vi "Remote Activate.vi"(8 "error in":errorcluster, 11 "Master Controller in":refnum<class "EMS User Interface.lvclass">) -> (0 "error out":errorcluster, 3 "Master Controller out":refnum<class "EMS User Interface.lvclass">)   [LabVIEW 2018, in "EMS User Interface Actor.lvlib" / "EMS User Interface.lvclass"]
uses:
  EMS User Interface.lvclass
  EMS User Interface.lvclass/EMS User Interface.ctl
  <vilib>/ActorFramework/Message Enqueuer/Message Enqueuer.lvclass/Message Enqueuer.ctl
  <vilib>/ActorFramework/Message Enqueuer/Enqueue.vi
  EMS Core/EMS Messages/Activate Init Msg/Activate Init Msg.lvclass
  C:/Program Files (x86)/National Instruments/LabVIEW 2018/vi.lib/ActorFramework/Message/Message.lvclass
  <vilib>/ActorFramework/Message Priority Queue/Priority Enqueue.vi
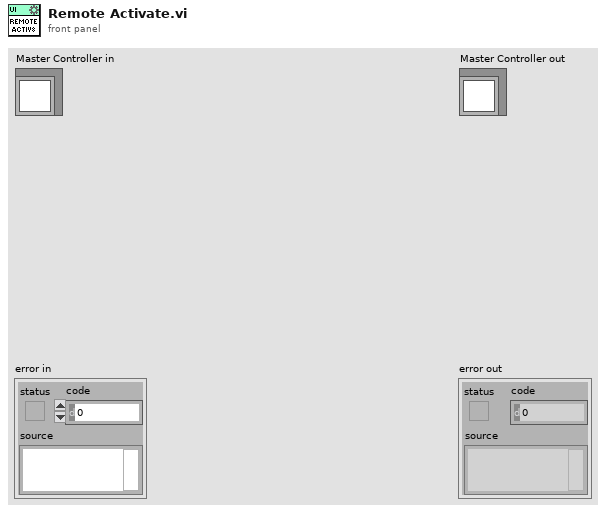
[diagram p1: front panel]
types:
  T1 = typedef "EMS Core.lvlib/EMS.lvclass/Microgrid State.ctl" = enum16{"Discovery", "Commissioning", "Activation", "Blackstart", "OnGrid", "OffGrid", "Island", "Resynchronization", "Manual", "Shutdown", "Stop"}
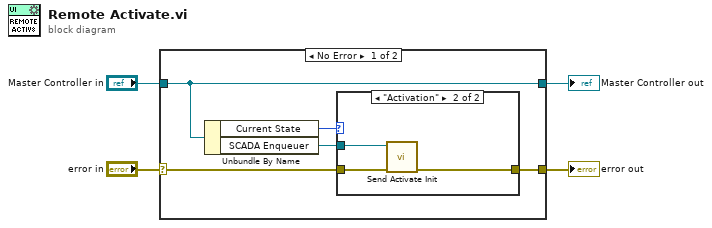
[diagram p0: block diagram]
diagram:
  n1 = case shown="No Error" "error in" {
    selector: "error in" -> [w6 w15]
    tunnel: [w5 w15] -> w2
    tunnel: [w9 w14] -> w1
    tunnel: "Master Controller in" -> [w9 w14]
    frame No Error {
      n2 = Unbundle By Name(w9) -> ("Current State"=w8:T1, "SCADA Enqueuer"=w7:refnum<class "Message Enqueuer.lvclass">)
      n3 = case shown="\"Activation\"" w8 {
        tunnel: w7 -> [_ w13]
        tunnel: [w10 w12] -> w5
        tunnel: w6 -> [w10 w11]
        frame "Discovery", Default {
        }
        frame "Activation" {
          n4 = call "Send Activate Init.vi"("error in (no error)"=w11, "Message Enqueuer"=w13) -> ("error out"=w12:errorcluster)  [unwired: 8 in, 1 out]
        }
      }
    }
    frame Error {
    }
  }
  "error out" <- w2
  "Master Controller out" <- w1
